vi "shutdown dispatcher.vi"(8 "error in":errorcluster, 11 "thread pool":refnum<class "thread pool.lvclass">) -> (0 "error out":errorcluster)   [LabVIEW 2014, in "thread pool.lvclass"]
uses:
  thread pool.lvclass
  task/strict executor reference.ctl
  thread pool.lvclass/thread pool.ctl
  results reporter/results reporter.lvclass
  task/task.lvclass
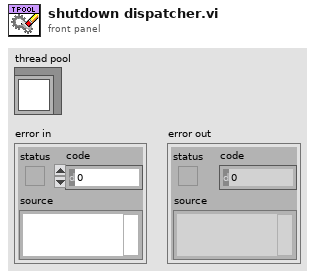
[diagram p1: front panel]
types:
  T1 = typedef "thread pool.lvclass/strict executor reference.ctl" = refnum<vi>
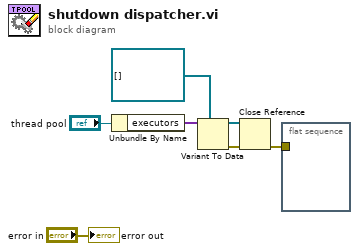
[diagram p0: block diagram]
diagram:
  n1 = Unbundle By Name("thread pool") -> ("executors"=w4:variant[])
  n2 = Variant To Data(type=T1[] [], Variant=w4) -> (data=w1:T1[], error out=w5:errorcluster)  [unwired: 1 in]
  n3 = Close Reference(reference=w1, error in (no error)=w5) -> (error out=w7:errorcluster)
  n4 = flat-sequence {
    tunnel: w7 -> [_]
    frame #0 {
    }
  }
  "error out" <- "error in"
